vi "Configure Serial Settings.vi"(0 "VISA resource name":refnum<visa-resource-name>, 1 "timeout (10sec)":u32=10000, 2 "termination char\n(0xA = '\\n' = LF)":u8=10 format="%.0x", 3 "Enable Termination\nChar (T)":bool=TRUE, 5 "baud rate (9600)":u32=9600, 7 "data bits (8)":u16=8 min=5 max=8 step=1, 9 "parity (0:none)":enum16{"None", "Odd", "Even", "Mark", "Space"}(ring), 11 "error in (no error)":errorcluster, 12 "stop bits (10: 1 bit)":u16(ring)=10 items=["1.0"=10, "1.5"=15, "2.0"=20], 13 "flow control (0:none)":u16(ring) items=["None", "XON/XOFF", "RTS/CTS", "XON/XOFF & RTS/CTS", "DTR/DSR", "XON/XOFF & DTR/DSR"]) -> (4 "VISA resource name out":refnum<visa-resource-name>, 6 "Interface Type":u16(ring)=1 items=["GPIB"=1, "VXI"=2, "GPIB-VXI"=3, "Serial"=4, "PXI"=5, "TCPIP"=6, "USB"=7, "FireWire"=9], 15 "error out":errorcluster)   [LabVIEW 2020, in "Utilities.lvlib"]
doc: "Configures serial settings for either Serial or TCP/IP interfaces."
uses:
  Utilities.lvlib
  <vilib>/Instr/_visa.llb/VISA Configure Serial Port (Instr).vi
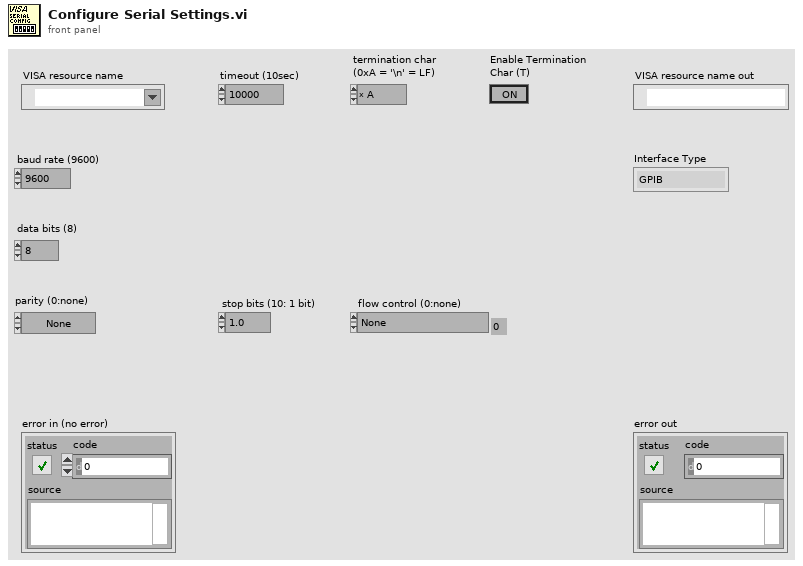
[diagram p1: front panel]
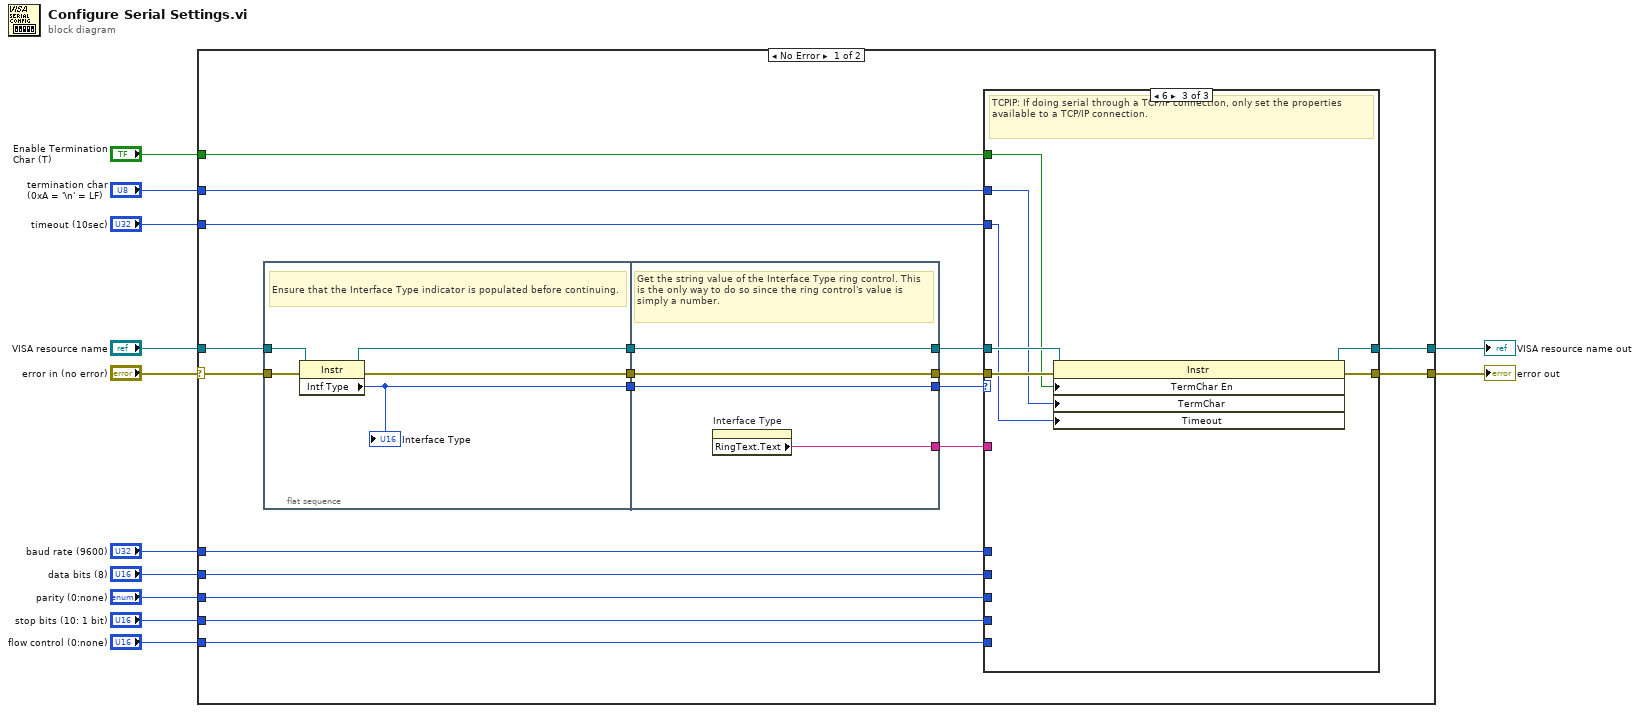
[diagram p0: block diagram]
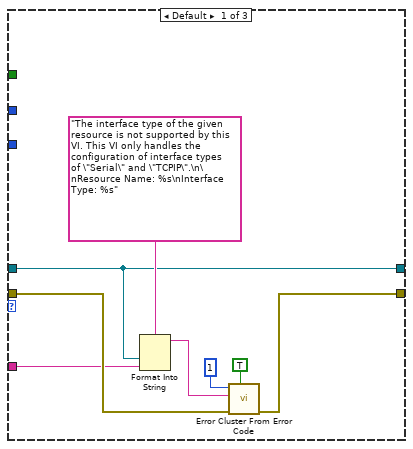
[diagram p2: hidden frame]
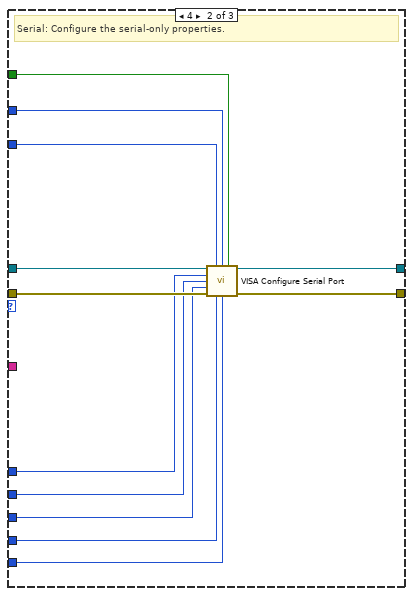
[diagram p3: hidden frame]
diagram:
  n1 = case shown="No Error" "error in (no error)" {
    selector: "error in (no error)" -> [w13 w68]
    tunnel: "VISA resource name" -> [w28 w69]
    tunnel: [w25 w69] -> w11
    tunnel: [w24 w68] -> w10
    tunnel: "Enable Termination\nChar (T)" -> [w23 _]
    tunnel: "termination char\n(0xA = '\\n' = LF)" -> [w22 _]
    tunnel: "timeout (10sec)" -> [w21 _]
    tunnel: "flow control (0:none)" -> [w20 _]
    tunnel: "stop bits (10: 1 bit)" -> [w19 _]
    tunnel: "parity (0:none)" -> [w18 _]
    tunnel: "data bits (8)" -> [w17 _]
    tunnel: "baud rate (9600)" -> [w16 _]
    frame No Error {
      n2 = flat-sequence {
        tunnel: w13 -> [w36]
        tunnel: w28 -> [w35]
        tunnel: [w34] -> w31
        tunnel: [w33] -> w30
        tunnel: [w32] -> w29
        tunnel: [w38] -> w26
        tunnel: [w39] -> w15
        tunnel: [w40] -> w27
        tunnel: w31 -> [w40]
        tunnel: w30 -> [w39]
        tunnel: w29 -> [w38]
        tunnel: [w37] -> w14
        frame #0 {
          # "Ensure that the Interface Type indicator is populated before continuing."
          n3 = property class="Instr"(reference=w35, error in=w36) -> (reference out=w32:refnum<visa-resource-name>, error out=w33:errorcluster, "Intf Type"=w34:u16)
          "Interface Type" <- w34
        }
        frame #1 {
          # "Get the string value of the Interface Type ring control. This is the only way to do so since the ring control's value is simply a number."
          n4 = property on="Interface Type" class="Ring (strict)"() -> ("RingText.Text"=w37:string)  [unwired: 2 in, 2 out]
        }
      }
      n5 = case shown="6" w27 {
        tunnel: w15 -> [w48 w60 w64]
        tunnel: w26 -> [w43 w59 w67]
        tunnel: [w43 w58 w66] -> w25
        tunnel: [w42 w57 w65] -> w24
        tunnel: w23 -> [_ w56 w63]
        tunnel: w22 -> [_ w55 w62]
        tunnel: w21 -> [_ w54 w61]
        tunnel: w20 -> [_ w53 _]
        tunnel: w19 -> [_ w52 _]
        tunnel: w18 -> [_ w51 _]
        tunnel: w17 -> [_ w50 _]
        tunnel: w16 -> [_ w49 _]
        tunnel: w14 -> [w47 _ _]
        frame Default {
          n6 = Format Into String(format string="The interface type of the given resource is not supported by this VI. This VI only handles the configuration of interface types of \"Serial\" and \"TCPIP\".\n\nResource Name: %s\nInterface Type: %s", w43, w47) -> (resulting string=w45:string)  [unwired: 2 in, 1 out]
          n7 = call <vilib>:"Error Cluster From Error Code.vi"("show call chain? (False)"=TRUE, "error in (no error)"=w48, "error message (\"\")"=w45, "error code (0)"=1) -> ("error out"=w42:errorcluster)  [unwired: 5 in]
        }
        frame 4 {
          # "Serial: Configure the serial-only properties."
          n8 = call-poly "VISA Configure Serial Port"("VISA resource name"=w59, "timeout (10sec)"=w54, "termination char\n(0xA = '\\n' = LF)"=w55, "Enable Termination\nChar (T)"=w56, "baud rate (9600)"=w49, "data bits (8)"=w50, "parity (0:none)"=w51, "error in (no error)"=w60, "stop bits (10: 1 bit)"=w52, "flow control (0:none)"=w53) -> ("VISA resource name out"=w58:refnum<visa-resource-name>, "error out"=w57:errorcluster)  [unwired: 4 in]
        }
        frame 6 {
          # "TCPIP: If doing serial through a TCP/IP connection, only set the properties available to a TCP/IP connection."
          n9 = property class="Instr"(reference=w67, error in=w64, "TermChar En"=w63, "TermChar"=w62, "Timeout"=w61) -> (reference out=w66:refnum<visa-resource-name>, error out=w65:errorcluster)
        }
      }
    }
    frame Error {
    }
  }
  "error out" <- w10
  "VISA resource name out" <- w11
